vi "OEE_SCREEN_2_update.vi"(8 "error_in":errorcluster, 11 "SCREEN_1":T2={"header_date"="-", "header_time"="-", "header_takt"="-", "header_shift"="-", "OP10_actual"="-", "OP10_rejects"="-", "OP10_quality_yeild"="-", "OP10_pace"="-", "OP20_actual"="-", "OP20_rejects"="-", "OP20_quality_yeild"="-", "OP20_pace"="-", "OP30_actual"="-", "OP30_rejects"="-", "OP30_quality_yeild"="-", "OP30_pace"="-", "OP40_actual"="-", "OP40_rejects"="-", "OP40_quality_yeild"="-", "OP40_pace"="-", "OP50_actual"="-", "OP50_rejects"="-", "OP50_quality_yeild"="-", "OP50_pace"="-", "OP60_actual"="-", "OP60_rejects"="-", "OP60_quality_yeild"="-", "OP60_pace"="-", "OP70_actual"="-", "OP70_rejects"="-", "OP70_quality_yeild"="-", "OP70_pace"="-", "OP80_actual"="-", "OP80_rejects"="-", "OP80_quality_yeild"="-", "OP80_pace"="-", "OP90_actual"="-", "OP90_rejects"="-", "OP90_quality_yeild"="-", "OP90_pace"="-", "OP100_actual"="-", "OP100_rejects"="-", "OP100_quality_yeild"="-", "OP100_pace"="-", "OP110_actual"="-", "OP110_rejects"="-", "OP110_quality_yeild"="-", "OP110_pace"="-", "OP120_actual"="-", "OP120_rejects"="-", "OP120_quality_yeild"="-", "OP120_pace"="-", "OP130_actual"="-", "OP130_rejects"="-", "OP130_quality_yeild"="-", "OP130_pace"="-", "OP10_header"="OP10", "OP20_header"="OP20", "OP30_header"="OP30", "OP40_header"="OP40", "OP50_header"="OP50", "OP60_header"="OP60", "OP70_header"="OP70", "OP80_header"="OP80", "OP90_header"="OP90", "OP100_header"="OP100", "OP110_header"="OP110", "OP120_header"="OP120", "OP130_header"="OP130", "additional_info"="", "bottleneck_OP"="-", "bottleneck_header"="LINE BOTTLENECK", "screen_1_header"="", "actual_header"="", "rejects_header"="", "FTTH_header"="", "pace_header"="", "actual_header"="", "rejects_header"="", "FTTH_header"="", "pace_header"=""}) -> (0 "error_out":errorcluster, 2 "SCREEN_2":T1={"header_part_no"="-", "header_customer"="-", "performance_percentage"="-", "performance_target"="-", "performance_actual"="-", "performance_header"="PERFORMANCE", "performance_target_header"="TARGET", "performance_actual_header"="ACTUAL", "screen_2_header"=""}, 3 "SCREEN_1":T2={"header_date"="-", "header_time"="-", "header_takt"="-", "header_shift"="-", "OP10_actual"="-", "OP10_rejects"="-", "OP10_quality_yeild"="-", "OP10_pace"="-", "OP20_actual"="-", "OP20_rejects"="-", "OP20_quality_yeild"="-", "OP20_pace"="-", "OP30_actual"="-", "OP30_rejects"="-", "OP30_quality_yeild"="-", "OP30_pace"="-", "OP40_actual"="-", "OP40_rejects"="-", "OP40_quality_yeild"="-", "OP40_pace"="-", "OP50_actual"="-", "OP50_rejects"="-", "OP50_quality_yeild"="-", "OP50_pace"="-", "OP60_actual"="-", "OP60_rejects"="-", "OP60_quality_yeild"="-", "OP60_pace"="-", "OP70_actual"="-", "OP70_rejects"="-", "OP70_quality_yeild"="-", "OP70_pace"="-", "OP80_actual"="-", "OP80_rejects"="-", "OP80_quality_yeild"="-", "OP80_pace"="-", "OP90_actual"="-", "OP90_rejects"="-", "OP90_quality_yeild"="-", "OP90_pace"="-", "OP100_actual"="-", "OP100_rejects"="-", "OP100_quality_yeild"="-", "OP100_pace"="-", "OP110_actual"="-", "OP110_rejects"="-", "OP110_quality_yeild"="-", "OP110_pace"="-", "OP120_actual"="-", "OP120_rejects"="-", "OP120_quality_yeild"="-", "OP120_pace"="-", "OP130_actual"="-", "OP130_rejects"="-", "OP130_quality_yeild"="-", "OP130_pace"="-", "OP10_header"="OP10", "OP20_header"="OP20", "OP30_header"="OP30", "OP40_header"="OP40", "OP50_header"="OP50", "OP60_header"="OP60", "OP70_header"="OP70", "OP80_header"="OP80", "OP90_header"="OP90", "OP100_header"="OP100", "OP110_header"="OP110", "OP120_header"="OP120", "OP130_header"="OP130", "additional_info"="", "bottleneck_OP"="-", "bottleneck_header"="LINE BOTTLENECK", "screen_1_header"="", "actual_header"="", "rejects_header"="", "FTTH_header"="", "pace_header"="", "actual_header"="", "rejects_header"="", "FTTH_header"="", "pace_header"=""})   [LabVIEW 2019]
uses:
  SCREEN_1/typedef/SCREEN_1.ctl
  typedef/SCREEN_2.ctl
  FGV/SQL_raw_data/FGV_OEE_SQL_raw_data.ctl
panel:
  # "OP"
  # "OP"
  # "OP"
  # "OP"
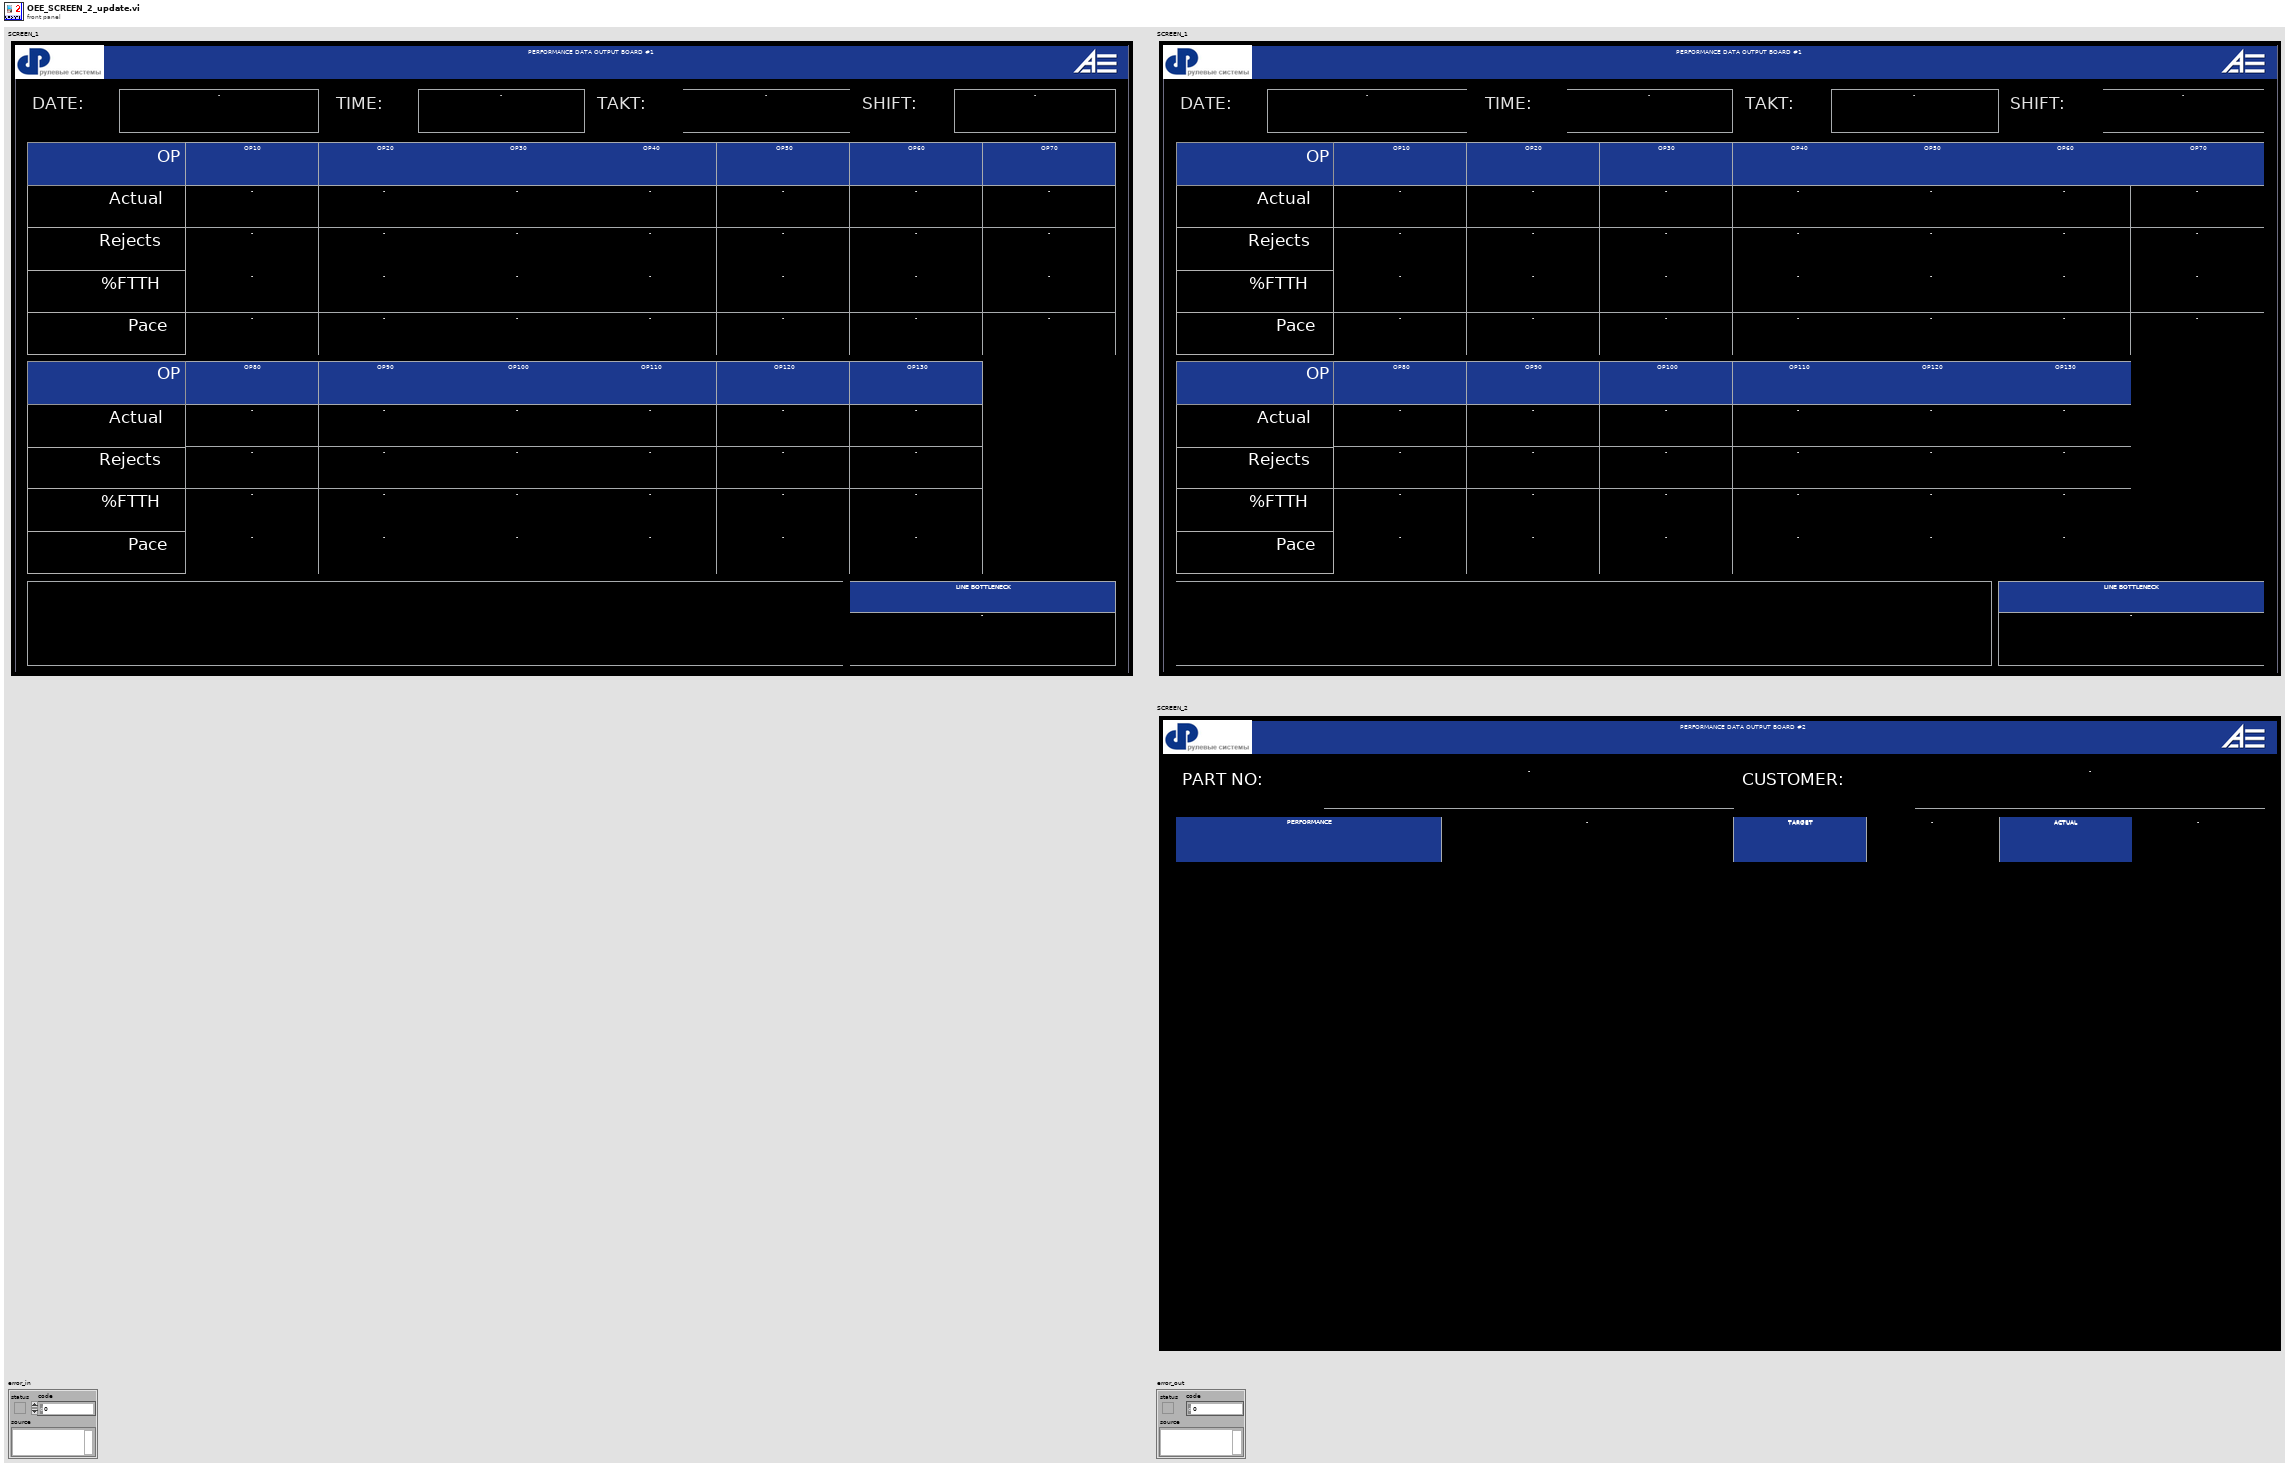
[diagram p1: front panel]
types:
  T1 = typedef "SCREEN_2.ctl" = cluster{"header_part_no":string, "header_customer":string, "performance_percentage":string, "performance_target":string, "performance_actual":string, "performance_header":string, "performance_target_header":string, "performance_actual_header":string, "screen_2_header":string}
  T2 = typedef "SCREEN_1.ctl" = cluster{"header_date":string, "header_time":string, "header_takt":string, "header_shift":string, "OP10_actual":string, "OP10_rejects":string, "OP10_quality_yeild":string, "OP10_pace":string, "OP20_actual":string, "OP20_rejects":string, "OP20_quality_yeild":string, "OP20_pace":string, "OP30_actual":string, "OP30_rejects":string, "OP30_quality_yeild":string, "OP30_pace":string, "OP40_actual":string, "OP40_rejects":string, "OP40_quality_yeild":string, "OP40_pace":string, "OP50_actual":string, "OP50_rejects":string, "OP50_quality_yeild":string, "OP50_pace":string, "OP60_actual":string, "OP60_rejects":string, "OP60_quality_yeild":string, "OP60_pace":string, "OP70_actual":string, "OP70_rejects":string, "OP70_quality_yeild":string, "OP70_pace":string, "OP80_actual":string, "OP80_rejects":string, "OP80_quality_yeild":string, "OP80_pace":string, "OP90_actual":string, "OP90_rejects":string, "OP90_quality_yeild":string, "OP90_pace":string, "OP100_actual":string, "OP100_rejects":string, "OP100_quality_yeild":string, "OP100_pace":string, "OP110_actual":string, "OP110_rejects":string, "OP110_quality_yeild":string, "OP110_pace":string, "OP120_actual":string, "OP120_rejects":string, "OP120_quality_yeild":string, "OP120_pace":string, "OP130_actual":string, "OP130_rejects":string, "OP130_quality_yeild":string, "OP130_pace":string, "OP10_header":string, "OP20_header":string, "OP30_header":string, "OP40_header":string, "OP50_header":string, "OP60_header":string, "OP70_header":string, "OP80_header":string, "OP90_header":string, "OP100_header":string, "OP110_header":string, "OP120_header":string, "OP130_header":string, "additional_info":string, "bottleneck_OP":string, "bottleneck_header":string, "screen_1_header":string, "actual_header":string, "rejects_header":string, "FTTH_header":string, "pace_header":string, "actual_header":string, "rejects_header":string, "FTTH_header":string, "pace_header":string}
  T3 = typedef "FGV_OEE_SQL_raw_data.ctl" = enum16{"initialize", "set_reference_name", "set_timestamp", "set_OK_NOK_count", "set_config_info", "set_pace", "set_availability", "set_hourly_ok_count", "set_targets", "get_all_info"}
  T4 = typedef "OEE_SQL_raw_data.ctl" = cluster{"reference_name":string, "data_timestamp":timestamp, "OK_NOK_count":string[][], "config_info":string[], "pace":string[][], "availability":string[], "hourly_ok_count":string[][], "shift_number":i8, "shift_start":i8, "shift_end":i8, "TAKT":u16, "FTTH_target":u16, "BOTTLENECK_station":string, "targets_hourly":u16[], "target_shift":u16}
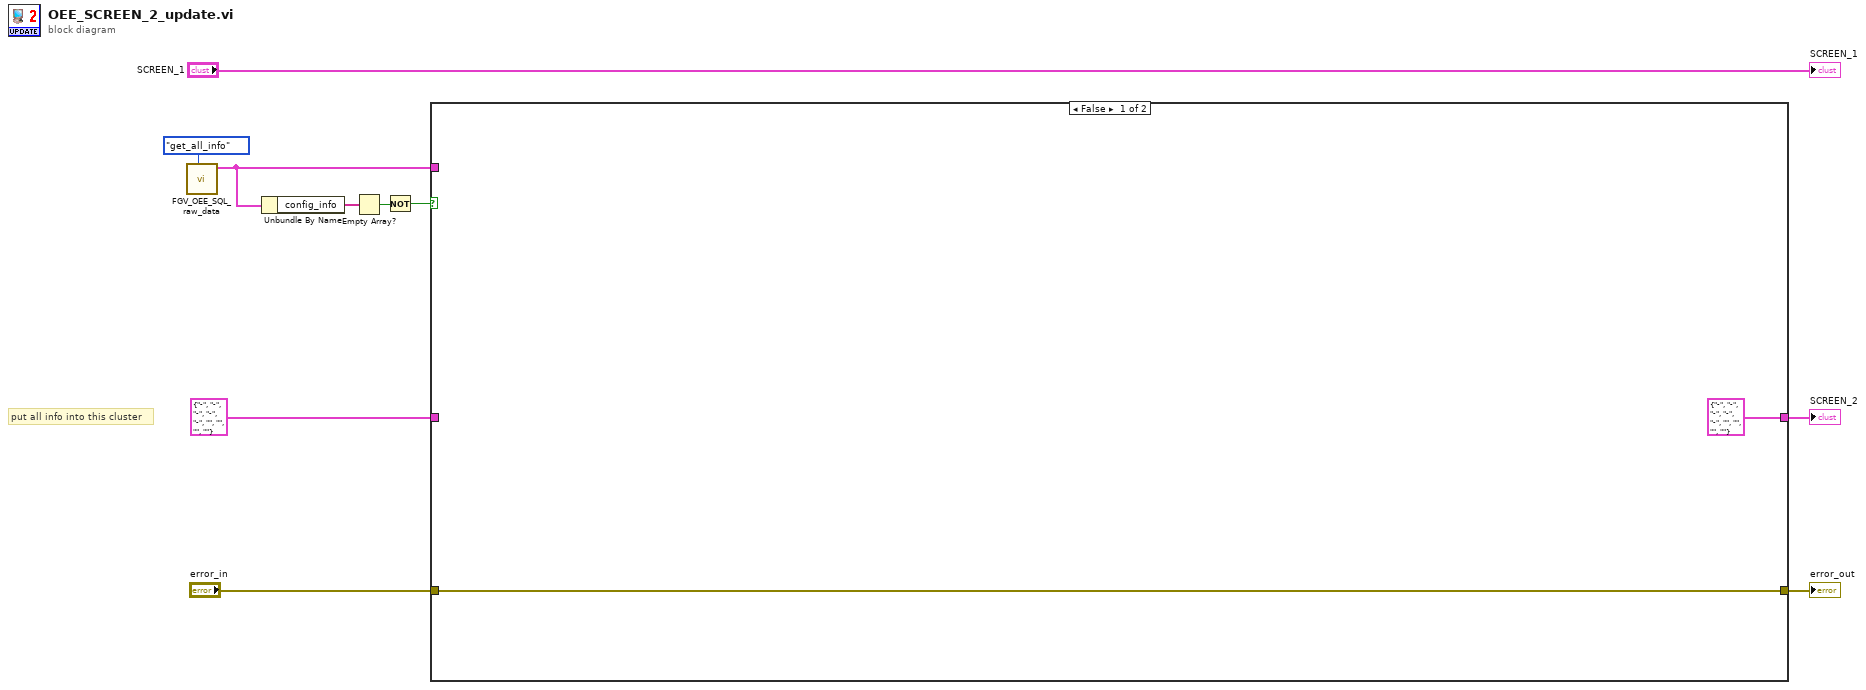
[diagram p0: block diagram]
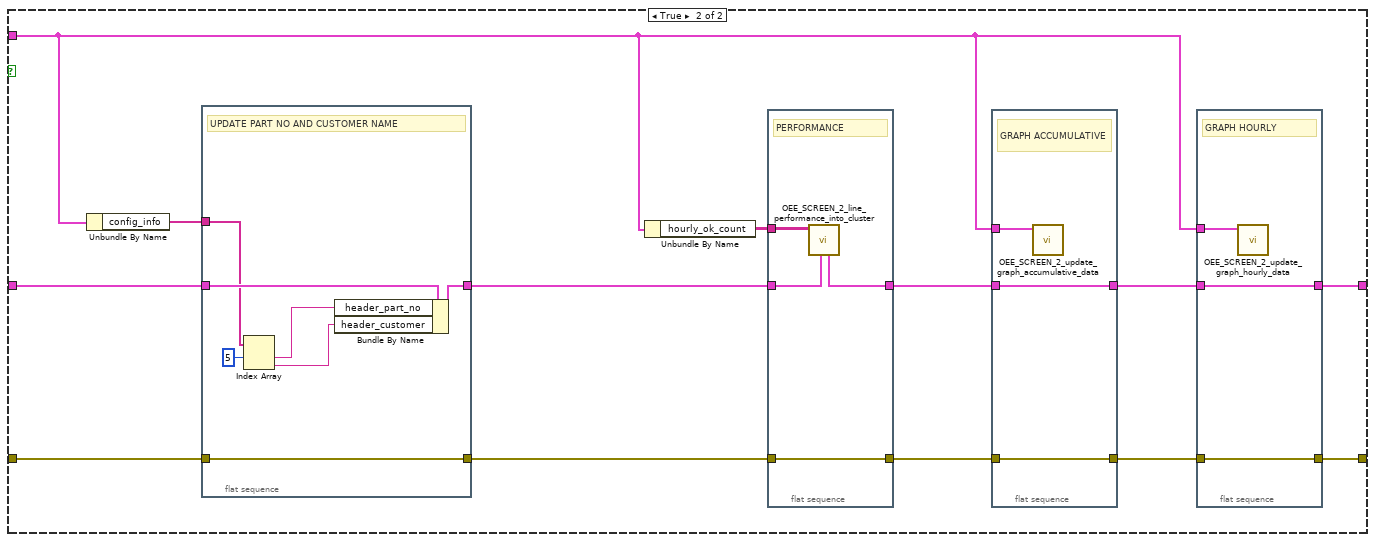
[diagram p2: hidden frame]
diagram:
  # "put all info into this cluster"
  n1 = call "FGV_OEE_SQL_raw_data.vi"("options"=FGV_OEE_SQL_raw_data."get_all_info") -> ("SQL_raw_data_out"=w2:T4)  [unwired: 9 in, 1 out]
  n2 = Unbundle By Name(w2) -> ("config_info"=w4:string[])
  n3 = Empty Array?(array=w4) -> (empty?=w3:bool)
  n4 = Not(x=w3) -> (.not. x?=w1:bool)
  n5 = case shown="False" w1 {
    tunnel: T1 {"header_part_no"="-", "header_customer"="-", "performance_percentage"="-", "performance_target"="-", "performance_actual"="-", "performance_header"="", "performance_target_header"="", "performance_actual_header"="", "screen_2_header"=""} ("SCREEN_2") -> [_ w25]
    tunnel: "error_in" -> [w11 w22]
    tunnel: w2 -> [_ w21]
    tunnel: [w11 w19] -> w7
    tunnel: [T1 {"header_part_no"="-", "header_customer"="-", "performance_percentage"="-", "performance_target"="-", "performance_actual"="-", "performance_header"="", "performance_target_header"="", "performance_actual_header"="", "screen_2_header"=""} ("SCREEN_2") w17] -> w6
    frame False {
    }
    frame True {
      n6 = Unbundle By Name(w21) -> ("config_info"=w24:string[])
      n7 = flat-sequence {
        tunnel: w25 -> [w42]
        tunnel: [w41] -> w16
        tunnel: w24 -> [w40]
        tunnel: w22 -> [w36]
        tunnel: [w36] -> w15
        frame #0 {
          # "UPDATE PART NO AND CUSTOMER NAME"
          n8 = Index Array(array=w40, index #1=5 ("index")) -> (element #1=w39:string, element #2=w38:string)  [unwired: 1 in]
          n9 = Bundle By Name(cluster=w42, "header_part_no"=w39, "header_customer"=w38) -> (w41:T1)
        }
      }
      n10 = Unbundle By Name(w21) -> ("hourly_ok_count"=w23:string[][])
      n11 = flat-sequence {
        tunnel: w16 -> [w35]
        tunnel: [w34] -> w14
        tunnel: w23 -> [w33]
        tunnel: w15 -> [w32]
        tunnel: [w32] -> w13
        frame #0 {
          # "PERFORMANCE"
          n12 = call "OEE_SCREEN_2_line_performance_into_cluster.vi"("SCREEN_2"=w35, "hourly_ok_count"=w33) -> ("SCREEN_2"=w34:T1)  [unwired: 9 in]
        }
      }
      n13 = flat-sequence {
        tunnel: w14 -> [w30]
        tunnel: w13 -> [w31]
        tunnel: [w31] -> w20
        tunnel: [w30] -> w18
        tunnel: w21 -> [w29]
        frame #0 {
          # "GRAPH ACCUMULATIVE"
          n14 = call "OEE_SCREEN_2_update_graph_accumulative_data.vi"("SQL_raw_data_out"=w29) -> ()  [unwired: 11 in]
        }
      }
      n15 = flat-sequence {
        tunnel: w20 -> [w28]
        tunnel: [w28] -> w19
        tunnel: w21 -> [w27]
        tunnel: w18 -> [w26]
        tunnel: [w26] -> w17
        frame #0 {
          # "GRAPH HOURLY"
          n16 = call "OEE_SCREEN_2_update_graph_hourly_data.vi"("SQL_raw_data_out"=w27) -> ()  [unwired: 11 in]
        }
      }
    }
  }
  "error_out" <- w7
  "SCREEN_2" <- w6
  "SCREEN_1" <- "SCREEN_1"
